vi "Subvi edge detector.vi"(8 "Input":bool) -> (2 "Output":bool)   [LabVIEW 2017]
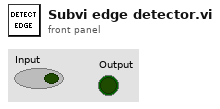
[diagram p1: front panel]
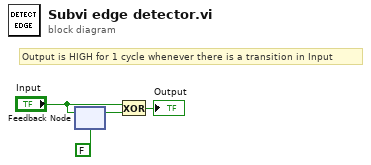
[diagram p0: block diagram]
diagram:
  # "Output is HIGH for 1 cycle whenever there is a transition in Input"
  n1 = feedback-in #1("Input") -> ()
  n2 = feedback #1(FALSE) -> (w4:bool)
  n3 = Exclusive Or(1:w4, 2:"Input") -> (0:→"Output":bool)
